vi "libssh2_channel_get_exit_status.vi"(8 "error in (no error)":errorcluster, 11 "channel":T1) -> (0 "error out":errorcluster, 3 "return value":i32)   [LabVIEW 2013, in "libssh2.lvlib"]
doc: "Gets the exit code raised by the process running on the remote host at the end of the named channel. Note that the exit status may not be available if the remote end has not yet set its status to closed."
uses:
  libssh2.lvlib
  Channel Refnum.ctl
  Global Settings.vi
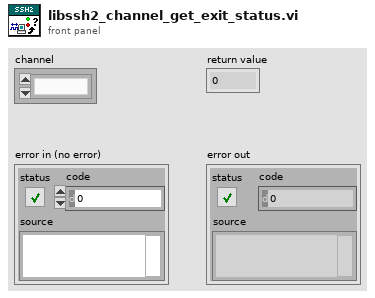
[diagram p1: front panel]
types:
  T1 = typedef "libssh2.lvlib/Channel Refnum.ctl" = refnum<k1>
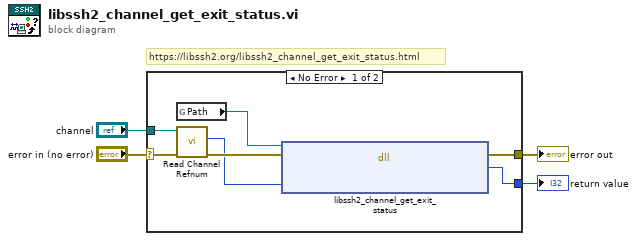
[diagram p0: block diagram]
diagram:
  # "https://libssh2.org/libssh2_channel_get_exit_status.html"
  n1 = case shown="No Error" "error in (no error)" {
    selector: "error in (no error)" -> [w6 w12]
    tunnel: [w11 _] -> w4
    tunnel: [w10 w12] -> w3
    tunnel: "channel" -> [w7 _]
    frame No Error {
      n2 = global read "Global Settings.vi" "Path"() -> (w5:path)
      n3 = call "Read Channel Refnum.vi"("error in (no error)"=w6, "channel"=w7) -> ("error out"=w9:errorcluster, "LIBSSH2_CHANNEL*"=w8:u64)  [unwired: 8 in]
      n4 = dll-call lib="C:/Users/pasca/source/repos/libssh2-labview/libssh2/libssh2**.*" fn="libssh2_channel_get_exit_status"(path in=w5, error in=w9, "channel"=w8) -> (error out=w10:errorcluster, "return value"=w11:i32)  [unwired: 2 in, 1 out]
    }
    frame Error {
    }
  }
  "return value" <- w4
  "error out" <- w3
